vi "createMissionWaypoints.vi"(8 "error in (no error)":errorcluster, 11 "Idle in":refnum<class "Idle.lvclass">) -> (0 "error out":errorcluster, 3 "Idle out":refnum<class "Idle.lvclass">)   [LabVIEW 2011, in "Idle.lvclass"]
doc: "Creates waypoint at current location, saves waypoint # so it can be deleted later, and saves current location. This is called on start."
uses:
  Idle.lvclass
  2 Globals/2 Global.vi
  Waypoint/Waypoint.lvclass
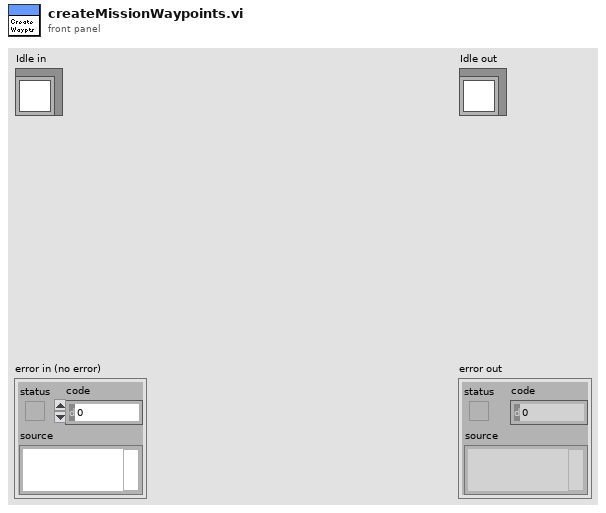
[diagram p1: front panel]
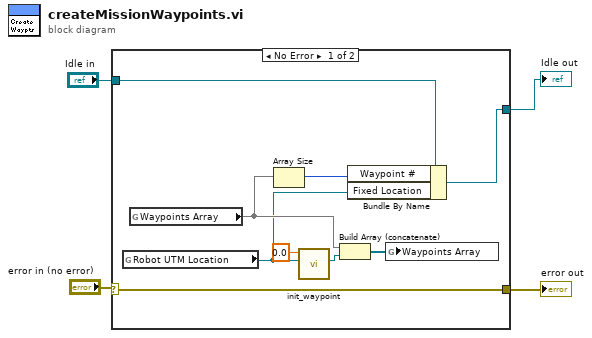
[diagram p0: block diagram]
diagram:
  n1 = case shown="No Error" "error in (no error)" {
    selector: "error in (no error)" -> [w13 w15]
    tunnel: [w13 w15] -> w3
    tunnel: "Idle in" -> [w8 w14]
    tunnel: [w7 w14] -> w1
    frame No Error {
      n2 = global read "2 Global.vi" "Robot UTM Location"() -> (w5:refnum<class "UTM_Location.lvclass">)
      n3 = global read "2 Global.vi" "Waypoints Array"() -> (w9)
      n4 = Array Size(array=w9) -> (size(s)=w6:i32)
      n5 = call "init_waypoint.vi"("Coords"=w5, "Tolerance (m)"=0.0) -> ("Waypoint Out"=w11:refnum<class "Waypoint.lvclass">)  [unwired: 9 in]
      n6 = Build Array (concatenate)(w9, w11) -> (w10:refnum<class "Waypoint.lvclass">[])
      n7 = Bundle By Name(cluster=w8, "Waypoint #"=w6, "Fixed Location"=w5) -> (w7:refnum<class "Idle.lvclass">)
      n8 = global write "2 Global.vi" "Waypoints Array"(w10) -> ()
    }
    frame Error {
    }
  }
  "error out" <- w3
  "Idle out" <- w1
